vi "Initialize DTC FIFOs.vi"(8 "error in":errorcluster, 11 "Simulated Addresses":T2[](array[typedef]) {"J1939 XNET Settings"."Name" format="%.0x"; "DM1 Data"."Data Reference" format="%.0x"; "DM1 Enable?"."Data Reference" format="%.0x"; "DM2 Data"."Data Reference" format="%.0x"; "DM2 Enable?"."Data Reference" format="%.0x"}) -> (0 "error out":errorcluster, 2 "Simulated Addresses LUT":variant, 3 "Simulated Addresses":T1[](array[typedef]) {"Simulated Addresses"."J1939 XNET Settings"."Name" format="%.0x"; "Simulated Addresses"."DM1 Data"."Data Reference" format="%.0x"; "Simulated Addresses"."DM1 Enable?"."Data Reference" format="%.0x"; "Simulated Addresses"."DM2 Data"."Data Reference" format="%.0x"; "Simulated Addresses"."DM2 Enable?"."Data Reference" format="%.0x"})   [LabVIEW 2013, in "J1939 Addon Engine.lvlib"]
uses:
  J1939 Addon Engine.lvlib
  Shared/Types/Compiled Simulated Settings.ctl
  Shared/Types/Monitor Settings.ctl
  <vilib>/NI Veristand/Custom Device API/Block Data Reference.ctl
  <vilib>/NI Veristand/Custom Device API/Data Reference.ctl
  Types/Simulated Settings.ctl
  Types/DTC FIFOs.ctl
  Shared/J1939 Addon Shared.lvlib
  <vilib>/NI Veristand/Custom Device API/Custom Device API.lvlib
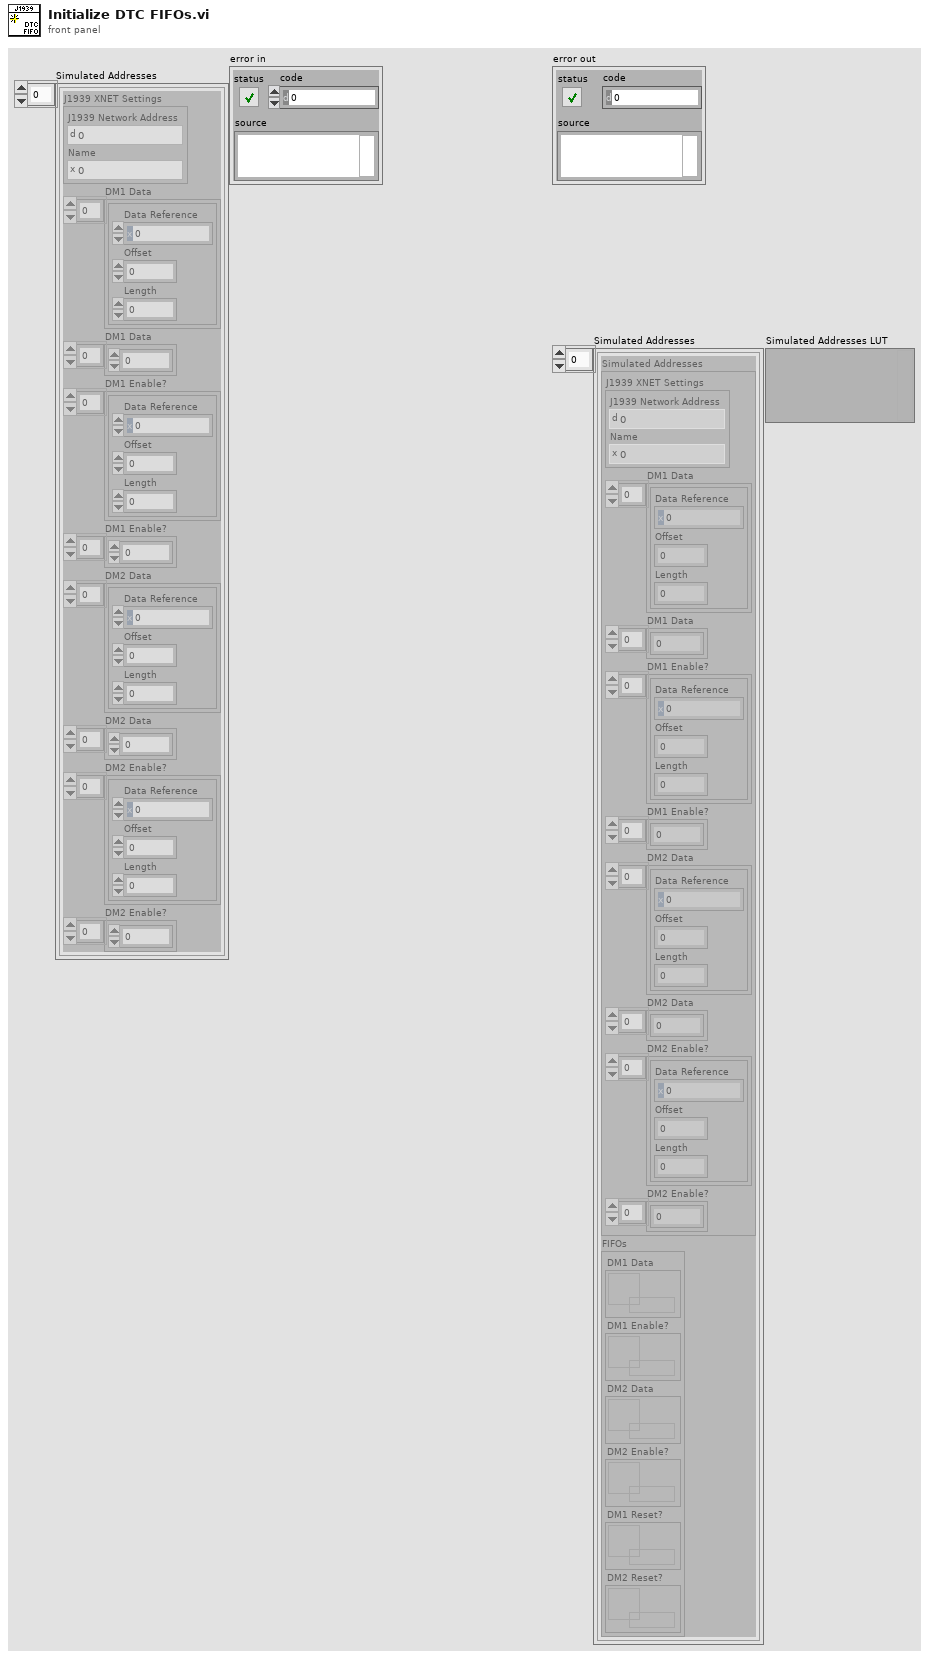
[diagram p1: front panel]
types:
  T1 = typedef "J1939 Addon Engine.lvlib/Simulated Settings.ctl" = cluster{"Simulated Addresses":T2, "FIFOs":T6}
  T2 = typedef "J1939 Addon Shared.lvlib/Compiled Simulated Settings.ctl" = cluster{"J1939 XNET Settings":T3, "DM1 Data":T4[], "DM1 Data":dbl[], "DM1 Enable?":T4[], "DM1 Enable?":dbl[], "DM2 Data":T4[], "DM2 Data":dbl[], "DM2 Enable?":T4[], "DM2 Enable?":dbl[]}
  T3 = typedef "J1939 Addon Shared.lvlib/Monitor Settings.ctl" = cluster{"J1939 Network Address":u8, "Name":u64}
  T4 = typedef "Custom Device API.lvlib/Block Data Reference.ctl" = cluster{"Data Reference":T5, "Offset":i32, "Length":i32}
  T5 = typedef "Custom Device API.lvlib/Data Reference.ctl" = i32
  T6 = typedef "J1939 Addon Engine.lvlib/DTC FIFOs.ctl" = cluster{"DM1 Data":refnum<k33>, "DM1 Enable?":refnum<k33>, "DM2 Data":refnum<k33>, "DM2 Enable?":refnum<k33>, "DM1 Reset?":refnum<k33>, "DM2 Reset?":refnum<k33>}
  T7 = cluster{"read mode":enum16{"polling", "blocking"}, "write mode":enum16{"polling", "blocking"}}
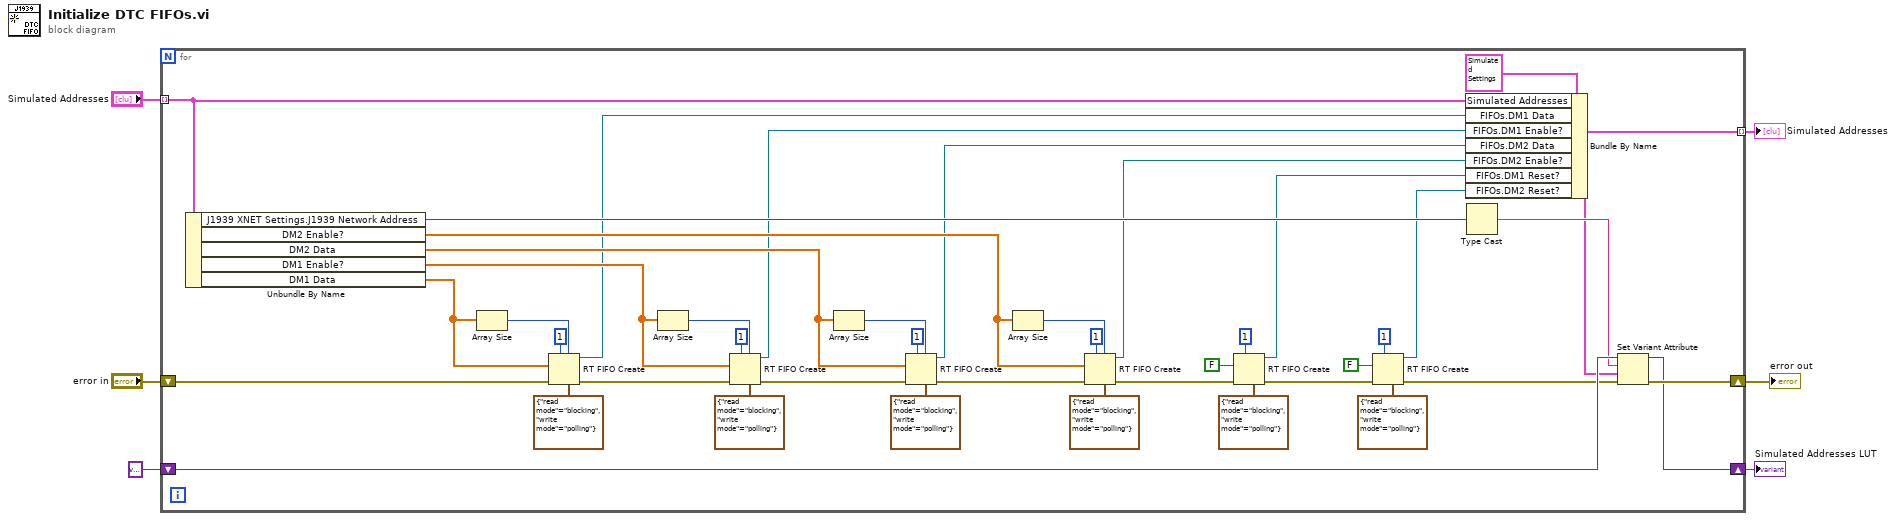
[diagram p0: block diagram]
diagram:
  n1 = for {
    tunnel: "Simulated Addresses" -> [w19] mode=indexing
    shift-right: [w29] -> w4
    shift-left: "error in" -> [w30]
    shift-right: [w25] -> w1
    shift-left: variant ("variant out") -> [w28]
    tunnel: [w18] -> w2 mode=indexing
    n2 = Unbundle By Name(w19) -> ("J1939 XNET Settings.J1939 Network Address"=w27:u8, "DM2 Enable?"=w31:dbl[], "DM2 Data"=w32:dbl[], "DM1 Enable?"=w33:dbl[], "DM1 Data"=w34:dbl[])
    n3 = Array Size(array=w34) -> (size(s)=w47:i32)
    n4 = RT FIFO Create(1:w34, 3:w30, 4:u32 1 ("size (10)"), 6:w47, 7:T7 {"read mode"=enum."blocking", "write mode"=enum."polling"} ("r/w modes (polling,polling)")) -> (8:w24:refnum<k33>, 11:w37:errorcluster)  [unwired: 3 in, 1 out]
    n5 = Array Size(array=w33) -> (size(s)=w46:i32)
    n6 = RT FIFO Create(1:w33, 3:w37, 4:u32 1 ("size (10)"), 6:w46, 7:T7 {"read mode"=enum."blocking", "write mode"=enum."polling"} ("r/w modes (polling,polling)")) -> (8:w23:refnum<k33>, 11:w36:errorcluster)  [unwired: 3 in, 1 out]
    n7 = Array Size(array=w32) -> (size(s)=w41:i32)
    n8 = RT FIFO Create(1:w32, 3:w36, 4:u32 1 ("size (10)"), 6:w41, 7:T7 {"read mode"=enum."blocking", "write mode"=enum."polling"} ("r/w modes (polling,polling)")) -> (8:w22:refnum<k33>, 11:w35:errorcluster)  [unwired: 3 in, 1 out]
    n9 = Array Size(array=w31) -> (size(s)=w40:i32)
    n10 = RT FIFO Create(1:w31, 3:w35, 4:u32 1 ("size (10)"), 6:w40, 7:T7 {"read mode"=enum."blocking", "write mode"=enum."polling"} ("r/w modes (polling,polling)")) -> (8:w21:refnum<k33>, 11:w15:errorcluster)  [unwired: 3 in, 1 out]
    n11 = RT FIFO Create(1:FALSE, 3:w15, 4:u32 1 ("size (10)"), 7:T7 {"read mode"=enum."blocking", "write mode"=enum."polling"} ("r/w modes (polling,polling)")) -> (8:w8:refnum<k33>, 11:w10:errorcluster)  [unwired: 4 in, 1 out]
    n12 = RT FIFO Create(1:FALSE, 3:w10, 4:u32 1 ("size (10)"), 7:T7 {"read mode"=enum."blocking", "write mode"=enum."polling"} ("r/w modes (polling,polling)")) -> (8:w7:refnum<k33>, 11:w9:errorcluster)  [unwired: 4 in, 1 out]
    n13 = Bundle By Name(cluster=T1 {"Simulated Addresses"={"J1939 XNET Settings"={"J1939 Network Address"=0, "Name"=0}, "DM1 Data"=[], "DM1 Data"=[], "DM1 Enable?"=[], "DM1 Enable?"=[], "DM2 Data"=[], "DM2 Data"=[], "DM2 Enable?"=[], "DM2 Enable?"=[]}, "FIFOs"={"DM1 Data"=refnum, "DM1 Enable?"=refnum, "DM2 Data"=refnum, "DM2 Enable?"=refnum, "DM1 Reset?"=refnum, "DM2 Reset?"=refnum}}, "Simulated Addresses"=w19, "FIFOs.DM1 Data"=w24, "FIFOs.DM1 Enable?"=w23, "FIFOs.DM2 Data"=w22, "FIFOs.DM2 Enable?"=w21, "FIFOs.DM1 Reset?"=w8, "FIFOs.DM2 Reset?"=w7) -> (w18:T1)
    n14 = Type Cast(x=w27) -> (*(type *) &x=w26:string)  [unwired: 1 in]
    n15 = Set Variant Attribute(Variant=w28, name=w26, value=w18, error in=w9) -> (Variant out=w25:variant, error out=w29:errorcluster)  [unwired: 1 out]
  }
  "error out" <- w4
  "Simulated Addresses" <- w2
  "Simulated Addresses LUT" <- w1
